vi "Register Messages.vi"(8 "error in (no error)":errorcluster, 10 "Messages Registration":T1, 11 "Remote Messaging Module in":refnum<class "Remote Messaging Module.lvclass">) -> (0 "error out":errorcluster, 3 "Remote Messaging Module out":refnum<class "Remote Messaging Module.lvclass">)   [LabVIEW 2020, in "Volatus.lvlib" / "Remote Messaging Module.lvclass"]
uses:
  Remote Messaging Module.lvclass
  Messages Registration.ctl
  MessageQ/MessageQ.lvclass
  Message Registration.ctl
  Remote Messaging Module.lvclass/Remote Messaging Module.ctl
  Type Handler.ctl
  <vilib>/Utility/miscctls.llb/LVMapReplaceAction.ctl
  Volatus.lvlib
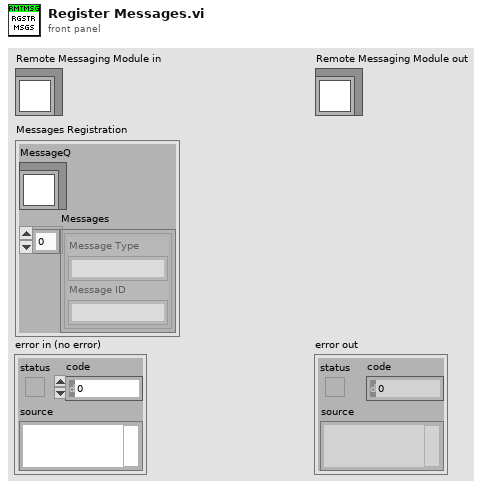
[diagram p1: front panel]
types:
  T1 = typedef "Volatus.lvlib/Messages Registration.ctl" = cluster{"MessageQ":refnum<class "MessageQ.lvclass">, "Messages":T2[]}
  T2 = typedef "Volatus.lvlib/Message Registration.ctl" = cluster{"Message Type":string, "Message ID":string}
  T3 = typedef "LVMapReplaceAction.ctl" = enum32{"Modify Entry only if found", "Add or Modify Entry", "Delete Entry"}
  T4 = typedef "Volatus.lvlib/Remote Messaging Module.lvclass/Type Handler.ctl" = cluster{"Msg ID":string, "MsgQ":refnum<class "MessageQ.lvclass">}
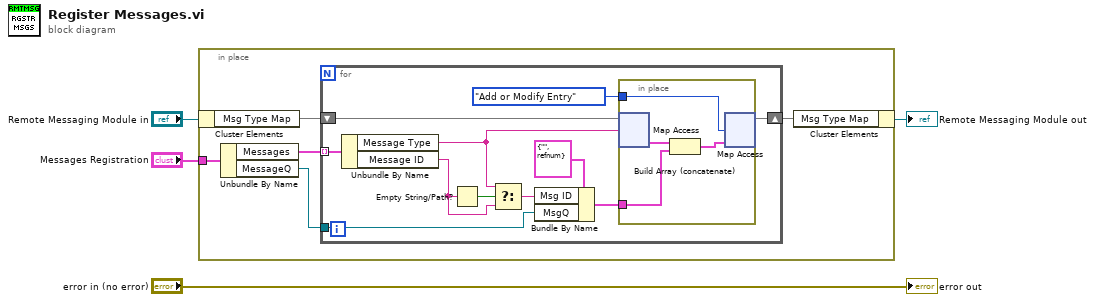
[diagram p0: block diagram]
diagram:
  n1 = in-place {
    in-place-border: "Messages Registration" -> [w9]
    n2 = in-place-cluster #1("Remote Messaging Module in") -> ("Msg Type Map"=w8:map{string, T4[]})
    n3 = Unbundle By Name(w9) -> ("Messages"=w7:T2[], "MessageQ"=w6:refnum<class "MessageQ.lvclass">)
    n4 = for {
      shift-right: [w10] -> w5
      shift-left: w8 -> [w14]
      tunnel: w7 -> [w20] mode=indexing
      tunnel: w6 -> [w15]
      n5 = Unbundle By Name(w20) -> ("Message Type"=w13:string, "Message ID"=w18:string)
      n6 = Empty String/Path?(string/path=w18) -> (empty?=w19:bool)
      n7 = Select(t=w13, s=w19, f=w18) -> (s? t:f=w16:string)
      n8 = Bundle By Name(cluster=T4 {"Msg ID"="", "MsgQ"=refnum} ("Type Handler"), "Msg ID"=w16, "MsgQ"=w15) -> (w12:T4)
      n9 = in-place {
        in-place-border: w12 -> [w23]
        in-place-border: LVMapReplaceAction."Add or Modify Entry" ("action") -> [w21]
        n10 = in-place-map #2(w14, w13) -> (w24:T4[])  [unwired: 1 in, 1 out]
        n11 = Build Array (concatenate)(w24, w23) -> (w22:T4[])
        n12 = in-place-map #2(w22, w21) -> (w10:map{string, T4[]})  [unwired: 2 out]
      }
    }
    n13 = in-place-cluster #1("Msg Type Map"=w5) -> (→"Remote Messaging Module out":refnum<class "Remote Messaging Module.lvclass">)
  }
  "error out" <- "error in (no error)"
